vi "Convert Package (VIPM to NIPM).vi"(6 "Category":string(combo)="Add-Ons", 8 "error in (no error)":errorcluster, 9 "LabVIEW version":string, 10 "Destination folder":path, 11 "Source VIPM package (.vip)":path) -> (0 "error out":errorcluster, 3 "Generated NIPM package (.nipkg)":path, 4 "Dependencies":T1)   [LabVIEW 2014, in "vipm-to-nipm-package-converter.lvlib"]
doc: "Converts a VIPM package (.vip) into a NIPM package (.nipkg) for a specific version of LabVIEW.\n\nINPUT(S):\n<b>Source VIPM package (.vip)</b>: Specifies the filepath of the source VIPM package (.vip) to convert. This VIPM package must be installed to the specified version of LabVIEW prior to running this VI.\n<b>Destination folder</b>: Specifies the destination folderpath to place the generated NIPM package(s) (.nipkg)\n<b>LabVIEW version</b>: Specifies the LabVIEW version for the NIPM package to support (\"14.0\", \"14.0 (64-bit)\", \"18.0\", \"18.0 (64-bit)\", etc)\n<b>Category</b>: (Optional) Specify the Category NIPM package attribute. The default is Add-Ons.\n\nOUTPUT(S):\n<b>Generated NIPM package (.nipkg)</b>: Specifies the filepath of the generated NIPM package (.nipkg)\n<b>Dependencies</b>: Outputs the source VIPM package's dependencies and the generated NIPM package's dependencies.\n\nDETAILS:\nThe generated NIPM package's attributes will inherit the VIPM package's name, display name, version, description, summary, vendor, URL, release notes, dependencies, and conflicts. The generated NIPM package does not support converting VIPM pre/post install/uninstall script VIs, and this VI will output a warning if script VI is detected in the VIPM package. Installing the generated NIPM package does not require the target computer to have VIPM Pro."
uses:
  vipm-to-nipm-package-converter.lvlib
  support/dependencies.ctl
  <vilib>/Utility/sysdir.llb/System Directory Type.ctl
  <vilib>/National Instruments/NIPM API (Beta)/NIPM_API.lvlib
panel:
  # "e.g. \"14.0\", \"14.0 (64-bit)\", \"18.0\", \"18.0 (64-bit)\""
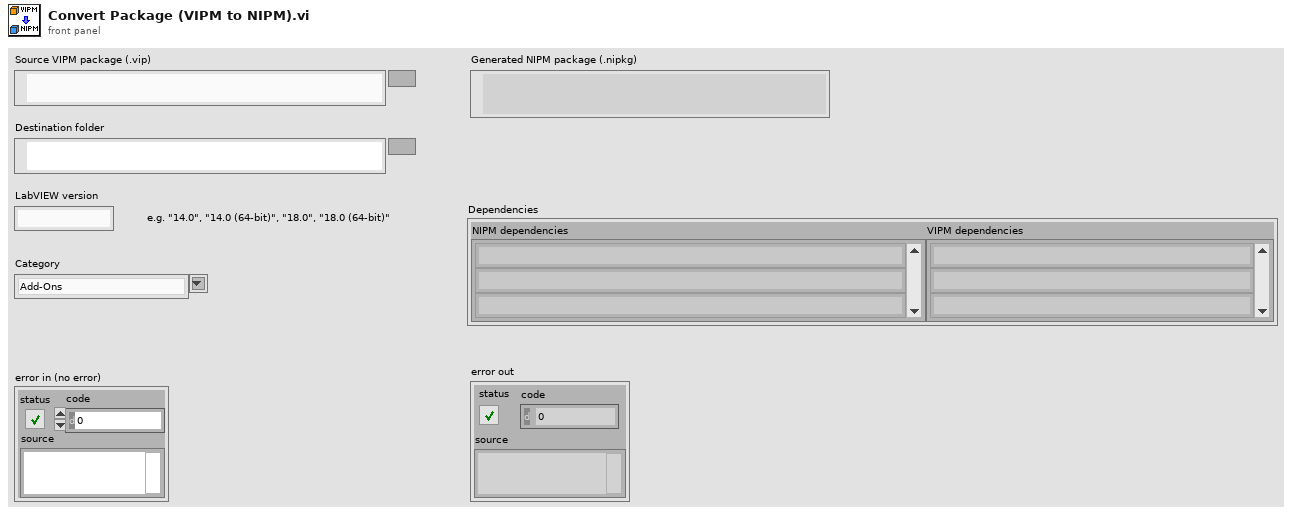
[diagram p1: front panel]
types:
  T1 = typedef "vipm-to-nipm-package-converter.lvlib/dependencies.ctl" = cluster{"NIPM dependencies":string[], "VIPM dependencies":string[]}
  T2 = enum16{"open", "replace", "create", "open or create", "replace or create", "replace or create with confirmation"}
  T3 = typedef "NIPM_API.lvlib/package attributes.ctl" = cluster{"Package Name":string, "Display name":string, "Version":string, "Display version":string, "Synopsis":string, "Description":string, "Maintainer":string, "Maintainer email address":string, "Category":string, "Homepage":string, "Release notes":string, "Depends":string[], "Recommends":string[], "Suggests":string[], "Conflicts":string[], "Provides":string[], "Replaces":string[], "Supplements":string[], "Enhances":string[], "Product":bool, "User visible":bool, "Installed size (KB)":u64, "Package filesize (bytes)":u64, "Architecture":string, "Agent":string, "MD5Checksum":string}
  T4 = typedef "System Directory Type.ctl" = i32
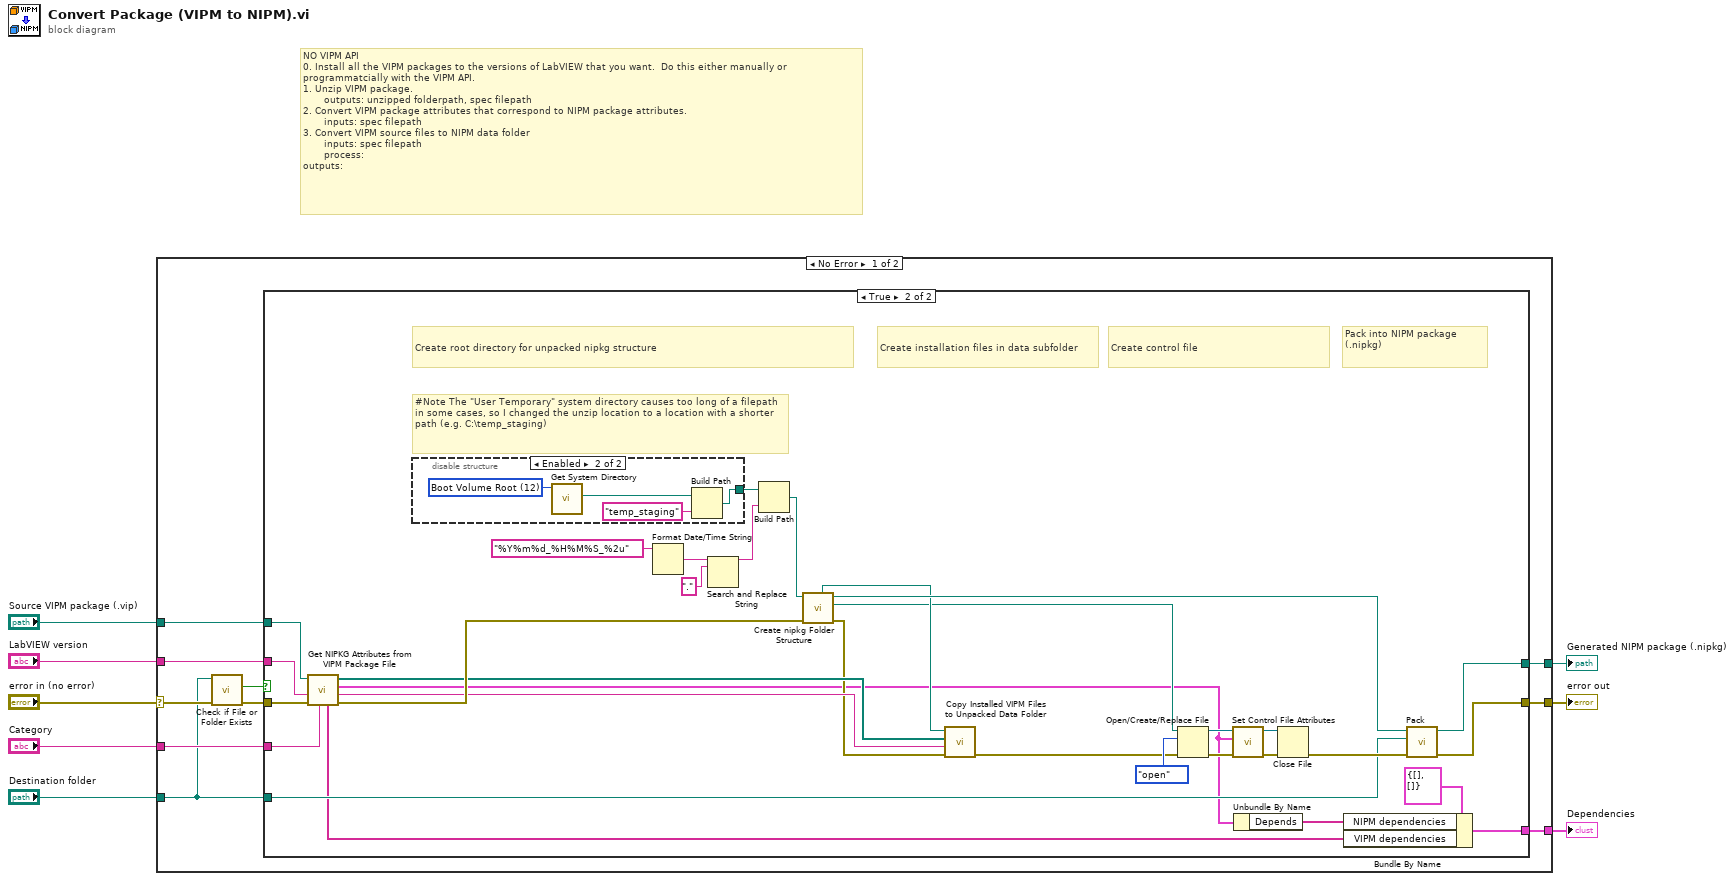
[diagram p0: block diagram]
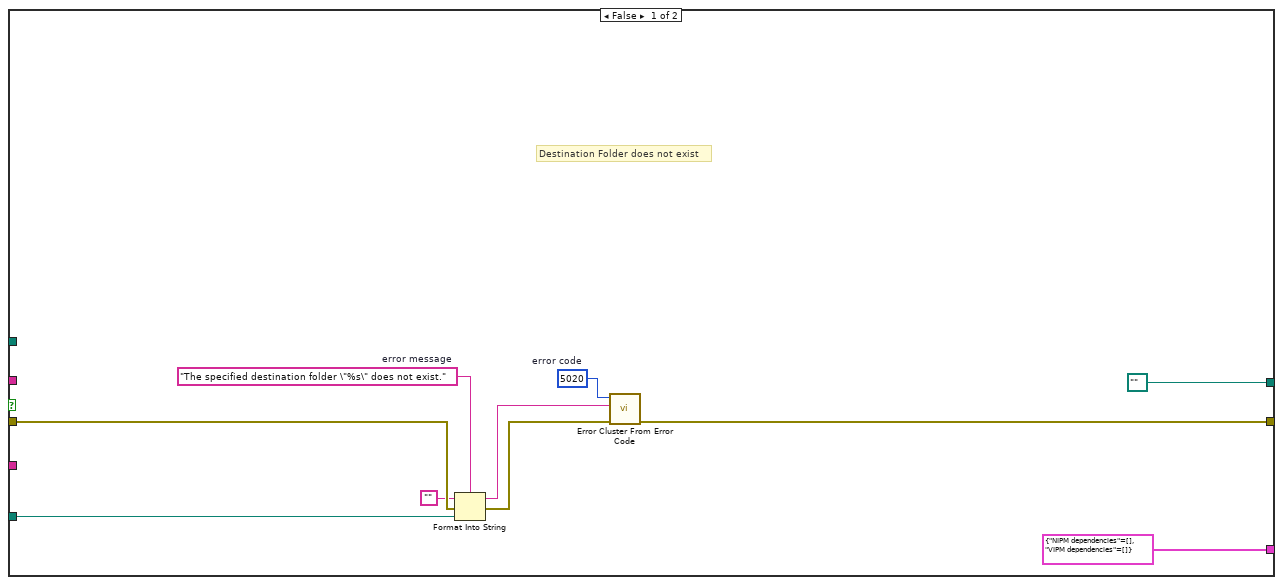
[diagram p2: hidden frame]
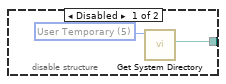
[diagram p3: hidden frame]
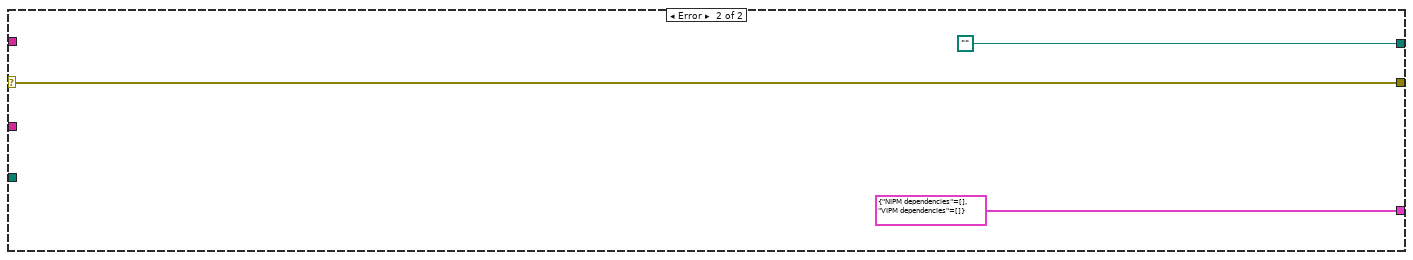
[diagram p4: hidden frame]
diagram:
  # "NO VIPM API\n0. Install all the VIPM packages to the versions of LabVIEW that you want.  Do this either manually or programmatcially with the VIPM API.\n1. Unzip VIPM package.\n       outputs: unzipped folderpath, spec filepath \n2. Convert VIPM package attributes that correspond to NIPM package attributes.\n       inputs: spec filepath\n3. Convert VIPM source files to NIPM data folder\n       inputs: spec filepath\n       process: \noutputs:"
  n1 = case shown="No Error" "error in (no error)" {
    selector: "error in (no error)" -> [w16 w69]
    tunnel: "Source VIPM package (.vip)" -> [w14 _]
    tunnel: "LabVIEW version" -> [w13 _]
    tunnel: "Category" -> [w18 _]
    tunnel: "Destination folder" -> [w11 _]
    tunnel: [w17 w69] -> w4
    tunnel: [w15 path ""] -> w2
    tunnel: [w9 T1 {"NIPM dependencies"=[], "VIPM dependencies"=[]} ("Dependencies")] -> w1
    frame No Error {
      n2 = call <vilib>:"Check if File or Folder Exists.vi"("error in (no error)"=w16, "path"=w11) -> ("error out"=w12:errorcluster, "file or folder exists?"=w10:bool)  [unwired: 7 in, 1 out]
      n3 = case shown="True" w10 {
        tunnel: w18 -> [_ w52]
        tunnel: [w21 w49] -> w17
        tunnel: [path "" ("package filepath") w48] -> w15
        tunnel: w14 -> [_ w47]
        tunnel: w13 -> [_ w42]
        tunnel: w12 -> [w26 w35]
        tunnel: w11 -> [w27 w34]
        tunnel: [T1 {"NIPM dependencies"=[], "VIPM dependencies"=[]} ("Dependencies") w30] -> w9
        frame False {
          w24 = "The specified destination folder \"%s\" does not exist."  # error message
          w28 = 5020  # error code
          # "Destination Folder does not exist"
          n4 = Format Into String(format string=w24, initial string="", error in=w26, w27) -> (resulting string=w22:string, error out=w25:errorcluster)
          n5 = call <vilib>:"Error Cluster From Error Code.vi"("error in (no error)"=w25, "error message (\"\")"=w22, "error code (0)"=w28) -> ("error out"=w21:errorcluster)  [unwired: 6 in]
        }
        frame True {
          # "#Note The \"User Temporary\" system directory causes too long of a filepath in some cases, so I changed the unzip location to a location with a shorter path (e.g. C:\\temp_staging)"
          # "Create control file"
          # "Pack into NIPM package\n(.nipkg)"
          # "Create installation files in data subfolder"
          # "Create root directory for unpacked nipkg structure"
          n6 = call "Get NIPKG Attributes from VIPM Package File.vi"("Category"=w52, "error in (no error)"=w35, "LabVIEW version"=w42, "Source VIPM package (.vip)"=w47) -> ("error out"=w46:errorcluster, "LabVIEW version out"=w40:string, "package attributes"=w33:T3, "VIPM Package Installed Filepaths"=w41:path[], "VIPM dependencies"=w31:string[])  [unwired: 3 in]
          n7 = disable-structure shown="Enabled" {
            disable-tunnel: [w61 w63] -> w60
            frame Disabled {
              w62 = T4 5 items=["User Home"=0, "User Desktop"=1, "User Documents"=2, "User Application Data"=3, "User Preferences"=4, "User Temporary"=5, "Public Documents"=6, "Public Application Data"=7, "Public Preferences"=8, "Public Cache"=13, "System Core Libraries"=9, "System Installed Libraries"=10, "Application Files"=11, "Boot Volume Root"=12] ("system directory type")
              n8 = call <vilib>:"Get System Directory.vi"("system directory type"=w62) -> ("system directory"=w61:path)  [unwired: 10 in]
            }
            frame Enabled {
              w66 = T4 12 items=["User Home"=0, "User Desktop"=1, "User Documents"=2, "User Application Data"=3, "User Preferences"=4, "User Temporary"=5, "Public Documents"=6, "Public Application Data"=7, "Public Preferences"=8, "Public Cache"=13, "System Core Libraries"=9, "System Installed Libraries"=10, "Application Files"=11, "Boot Volume Root"=12] ("system directory type")
              n9 = call <vilib>:"Get System Directory.vi"("system directory type"=w66) -> ("system directory"=w65:path)  [unwired: 10 in]
              n10 = Build Path(base path=w65, name or relative path="temp_staging") -> (appended path=w63:path)
            }
          }
          n11 = Format Date/Time String(time format string (%c)="%Y%m%d_%H%M%S_%2u") -> (date/time string=w44:string)  [unwired: 2 in]
          n12 = Search and Replace String(input string=w44, search string=".") -> (result string=w43:string)  [unwired: 6 in, 3 out]
          n13 = Build Path(base path=w60, name or relative path=w43) -> (appended path=w53:path)
          n14 = call "Create nipkg Folder Structure.vi"("error in (no error)"=w46, "target folder"=w53) -> ("error out"=w38:errorcluster, "control filepath"=w36:path, "nipkg unpacked folder"=w50:path, "data folderpath"=w37:path)  [unwired: 5 in, 1 out]
          n15 = call "Copy Installed VIPM Files to Unpacked Data Folder.vi"("error in (no error)"=w38, "LabVIEW version"=w40, "VIPM Package Installed Filepaths"=w41, "Unpacked Data Folder"=w37) -> ("error out"=w39:errorcluster)  [unwired: 6 in, 1 out]
          n16 = Open/Create/Replace File(file path (use dialog)=w36, error in=w39, operation (0:open)=T2."open") -> (refnum out=w57:refnum<file>, error out=w58:errorcluster)  [unwired: 3 in, 1 out]
          n17 = call <vilib>:"Set Control File Attributes.vi"("error in (no error)"=w58, "package attributes"=w33, "control file refnum in"=w57) -> ("error out"=w55:errorcluster, "control file refnum out"=w54:refnum<file>)  [unwired: 7 in]
          n18 = Unbundle By Name(w33) -> ("Depends"=w32:string[])
          n19 = Close File(refnum=w54, error in=w55) -> (error out=w51:errorcluster)  [unwired: 1 out]
          n20 = Bundle By Name(cluster=T1 {"NIPM dependencies"=[], "VIPM dependencies"=[]} ("Dependencies"), "NIPM dependencies"=w32, "VIPM dependencies"=w31) -> (w30:T1)
          n21 = call <vilib>:"Pack.vi"("error in"=w51, "destination folder"=w34, "source folder"=w50) -> ("error out"=w49:errorcluster, "package filepath"=w48:path)  [unwired: 7 in]
        }
      }
    }
    frame Error {
    }
  }
  "Generated NIPM package (.nipkg)" <- w2
  "error out" <- w4
  "Dependencies" <- w1
